vi "Auto Add Device Data Model.vi"(8 "error in":errorcluster, 10 "unit ID":u8, 11 "Super Data Model in":refnum<class "Super Data Model.lvclass">) -> (0 "error out":errorcluster, 2 "device data model":refnum<class "Standard Data Model.lvclass">, 3 "Super Data Model out":refnum<class "Super Data Model.lvclass">)   [LabVIEW 2013, in "Modbus Library - Advance.lvlib" / "Super Data Model.lvclass"]
uses:
  Super Data Model.lvclass
  Standard Data Model/Standard Data Model.lvclass
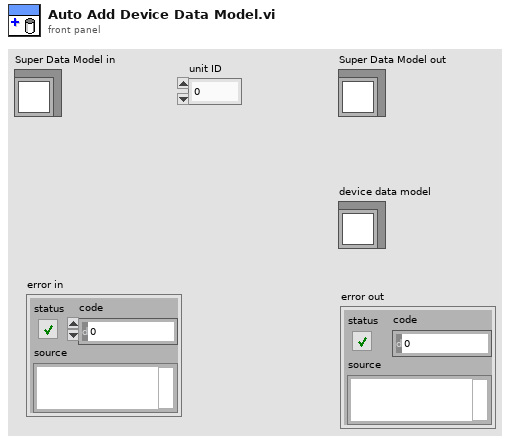
[diagram p1: front panel]
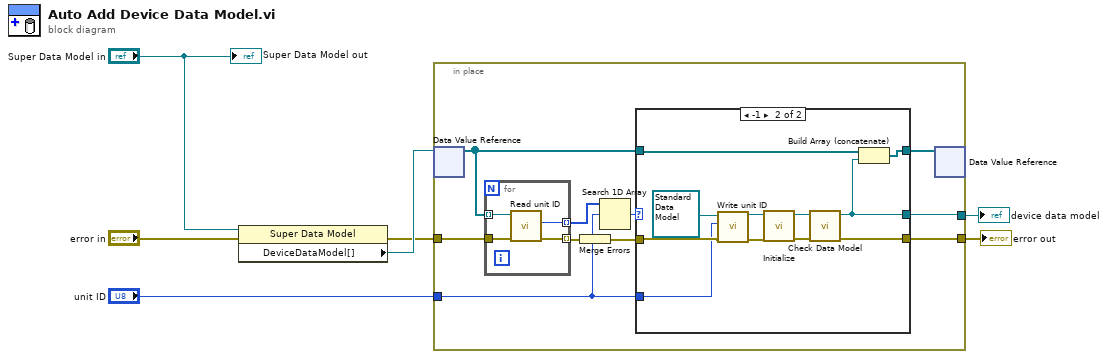
[diagram p0: block diagram]
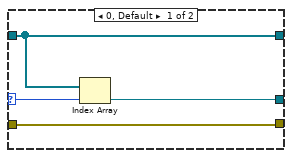
[diagram p2: hidden frame]
diagram:
  n1 = property class="Super Data Model"(reference="Super Data Model in", error in="error in") -> (error out=w4:errorcluster, "DeviceDataModel[]"=w6:refnum<data-value>)  [unwired: 1 out]
  n2 = in-place {
    in-place-border: "unit ID" -> [w9]
    in-place-border: w4 -> [w13]
    in-place-border: [w12] -> w1
    in-place-border: [w8] -> w2
    n3 = in-place-dvr #1(w6) -> (w15:refnum<class "Standard Data Model.lvclass">[])  [unwired: 1 out]
    n4 = for {
      tunnel: w15 -> [w36] mode=indexing
      tunnel: [w35] -> w17 mode=indexing
      tunnel: [w34] -> w11 mode=indexing
      tunnel: w13 -> [w33]
      n5 = call-dynamic "Read unit ID.vi"("error in (no error)"=w33, "Standard Data Model in"=w36) -> ("error out"=w34:errorcluster, "unit ID"=w35:u8)  [unwired: 7 in, 1 out]
    }
    n6 = Merge Errors(w11) -> (w10:errorcluster)
    n7 = Search 1D Array(1D array=w17, element=w9) -> (index of element=w16:i32)  [unwired: 1 in]
    n8 = case shown="-1" w16 {
      selector: w16 -> [w20 _]
      tunnel: w15 -> [w21 w25]
      tunnel: [w21 w23] -> w14
      tunnel: [w19 w26] -> w12
      tunnel: w10 -> [w19 w29]
      tunnel: w9 -> [_ w24]
      tunnel: [w18 w22] -> w8
      frame 0, Default {
        n9 = Index Array(array=w21, index=w20) -> (element=w18:refnum<class "Standard Data Model.lvclass">)
      }
      frame -1 {
        n10 = call-dynamic "Write unit ID.vi"("error in (no error)"=w29, "unit ID"=w24, "Standard Data Model in"=refnum<class "Standard Data Model.lvclass"> refnum ("device data model in")) -> ("error out"=w28:errorcluster, "Standard Data Model out"=w27:refnum<class "Standard Data Model.lvclass">)  [unwired: 7 in]
        n11 = call-dynamic "Initialize.vi"("error in"=w28, "device data model in"=w27) -> ("error out"=w32:errorcluster, "device data model out"=w31:refnum<class "Standard Data Model.lvclass">)  [unwired: 8 in]
        n12 = call-dynamic "Check Data Model.vi"("error in"=w32, "device data model in"=w31) -> ("error out"=w26:errorcluster, "device data model out"=w22:refnum<class "Standard Data Model.lvclass">)  [unwired: 8 in]
        n13 = Build Array (concatenate)(w25, w22) -> (w23:refnum<class "Standard Data Model.lvclass">[])
      }
    }
    n14 = in-place-dvr #1(w14) -> ()  [unwired: 2 out]
  }
  "error out" <- w1
  "device data model" <- w2
  "Super Data Model out" <- "Super Data Model in"
